vi "WPI_GyroXRS450_SPI_GetAngle.vi"(8 "error in":errorcluster, 11 "GyroDevRef":T1={"DevStatus"={"status"=FALSE, "code"=0, "source"=""}, "Analog Channel"=enum."AI 0", "Gain (VoltsPerDegree/Second)"=0.0, "Gyro Type"=enum."Analog", "Handle"=0, "SPI Bus"=enum."Invalid", "Device Found"=FALSE, "Sample Rate"=1.0, "Calibrate On Open"=FALSE, "Offset"=0.0} {"Sample Rate" min=0.25 max=100.0 step=0.25}) -> (0 "error out":errorcluster, 1 "Angular Rate":dbl, 2 "Angle":dbl, 3 "GyroDevRef":T1={"DevStatus"={"status"=FALSE, "code"=0, "source"=""}, "Analog Channel"=enum."AI 0", "Gain (VoltsPerDegree/Second)"=0.0, "Gyro Type"=enum."Analog", "Handle"=0, "SPI Bus"=enum."Invalid", "Device Found"=FALSE, "Sample Rate"=1.0, "Calibrate On Open"=FALSE, "Offset"=0.0} {"Sample Rate" min=0.25 max=100.0 step=0.25}, 4 "Calibrated?":bool)   [LabVIEW 2017]
doc: "Returns the angle, in degrees from the original heading, that the robot is currently facing.\n\nThis software is licensed. Open the labview\\readme\\WPI Robotics Library Open Source License.txt file for more information."
uses:
  <vilib>/Rock Robotics/WPI/Gyro/WPI_GyroDevRef.ctl
  <vilib>/Rock Robotics/SystemInterfaces/AI/FPGA_AIChannel.ctl
  <vilib>/Rock Robotics/SystemInterfaces/spilib/spi_bus.ctl
panel:
  # "Analog"
  # "XRS"
  # "Analog"
  # "XRS"
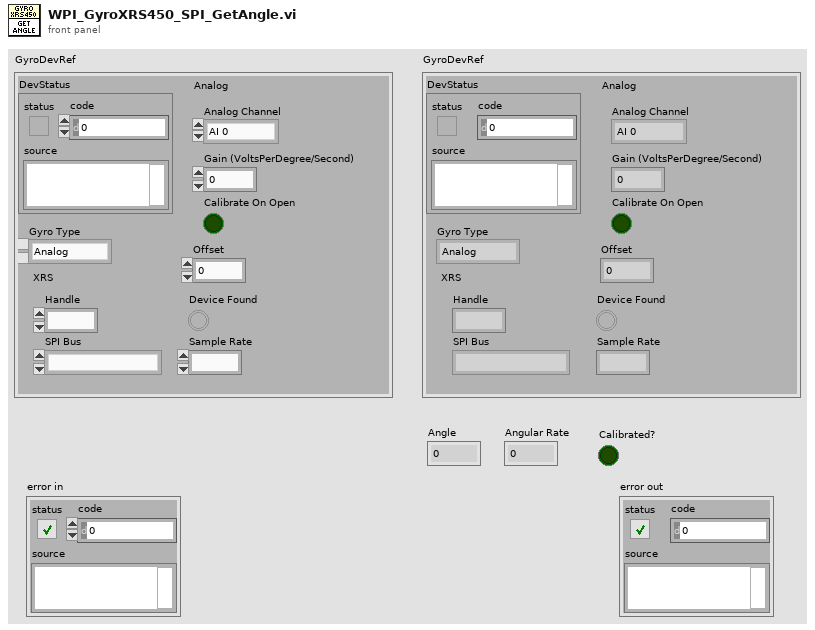
[diagram p1: front panel]
types:
  T1 = typedef "WPI_GyroDevRef.ctl" = cluster{"DevStatus":errorcluster, "Analog Channel":T2, "Gain (VoltsPerDegree/Second)":dbl, "Gyro Type":enum16{"Analog", "XRS450"}, "Handle":i32, "SPI Bus":T3, "Device Found":bool, "Sample Rate":dbl, "Calibrate On Open":bool, "Offset":dbl}
  T2 = typedef "FPGA_AIChannel.ctl" = enum8{"AI 0", "AI 1", "AI 2", "AI 3", "AI MXP 0", "AI MXP 1", "AI MXP 2", "AI MXP 3", "Invalid"}
  T3 = typedef "spi_bus.ctl" = enum16{"SPI On-Board, CS0", "SPI On-Board, CS1", "SPI On-Board, CS2", "SPI On-Board, CS3", "SPI MXP", "Invalid"}
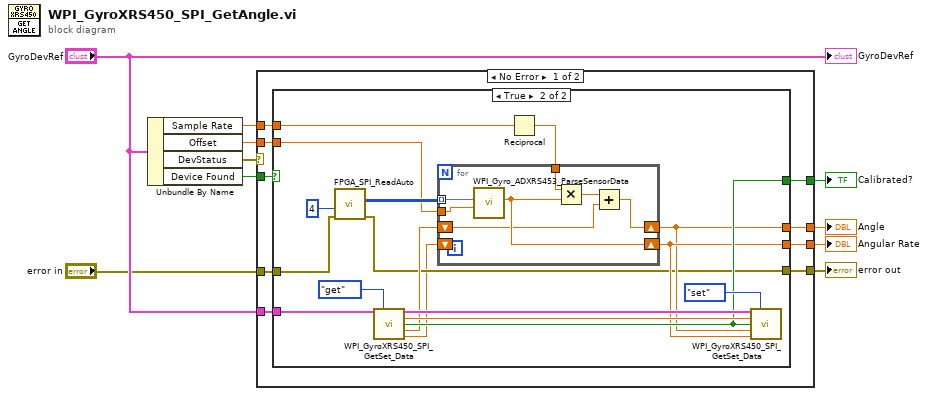
[diagram p0: block diagram]
diagram:
  n1 = Unbundle By Name("GyroDevRef") -> ("Sample Rate"=w10:dbl, "Offset"=w6:dbl, "DevStatus"=w2:errorcluster, "Device Found"=w1:bool)
  n2 = case shown="No Error" w2 {
    selector: w2 -> [_ w45]
    tunnel: w10 -> [w19 _]
    tunnel: "GyroDevRef" -> [w18 _]
    tunnel: [w17 _] -> w8
    tunnel: [w16 _] -> w7
    tunnel: w6 -> [w15 _]
    tunnel: [w14 _] -> w5
    tunnel: "error in" -> [w13 _]
    tunnel: [w12 w45] -> w3
    tunnel: w1 -> [w11 _]
    frame No Error {
      n3 = case shown="True" w11 {
        tunnel: w19 -> [_ w22]
        tunnel: w18 -> [_ w37]
        tunnel: [_ w30] -> w17
        tunnel: [_ w29] -> w16
        tunnel: w15 -> [_ w28]
        tunnel: [_ w26] -> w14
        tunnel: w13 -> [w20 w25]
        tunnel: [w20 w24] -> w12
        frame False {
        }
        frame True {
          n4 = call <vilib>:"FPGA_SPI_ReadAuto.vi"("error in (no error)"=w25, "Bytes per Sample"=u32 4) -> ("error out"=w24:errorcluster, "Data"=w32:u8[][])  [unwired: 8 in]
          n5 = call <vilib>:"WPI_GyroXRS450_SPI_GetSet_Data.vi"("GyroDeviceRef"=w37, "Operation"=enum16{"set", "get"}."get") -> ("GyroDeviceRef"=w34:T1, "Offset"=w33:dbl, "Calibrated?"=w30:bool, "Angle"=w27:dbl, "Rate"=w23:dbl)  [unwired: 9 in]
          n6 = Reciprocal(x=w22) -> (1/x=w21:dbl)
          n7 = for {
            tunnel: w32 -> [w44] mode=indexing
            tunnel: w28 -> [w43]
            shift-right: [w38] -> w26
            shift-left: w27 -> [w39]
            tunnel: w21 -> [w40]
            shift-right: [w42] -> w29
            shift-left: w23 -> [_]
            # "Offset Calibration"
            n8 = call <vilib>:"WPI_Gyro_ADXRS453_ParseSensorData.vi"("Offset"=w43, "Data"=w44) -> ("Angular Rate (deg/sec)"=w42:dbl)  [unwired: 7 in, 2 out]
            n9 = Multiply(x=w40, y=w42) -> (x*y=w41:dbl)
            n10 = Add(x=w41, y=w39) -> (x+y=w38:dbl)
          }
          n11 = call <vilib>:"WPI_GyroXRS450_SPI_GetSet_Data.vi"("GyroDeviceRef"=w34, "Operation"=enum16{"set", "get"}."set", "Offset"=w33, "Calibrated"=w30, "Angle"=w26, "Rate"=w29) -> ()  [unwired: 5 in, 5 out]
        }
      }
    }
    frame Error {
    }
  }
  "Angle" <- w5
  "error out" <- w3
  "Calibrated?" <- w8
  "Angular Rate" <- w7
  "GyroDevRef" <- "GyroDevRef"
